vi "get_erbumen_sp_gonghao.vi"(2 "juese":string, 4 "gonghao":string) -> (0 "sp":string[][](array[string]), 1 "error":errorcluster caption="error out 10")   [LabVIEW 2017, in "Lib_code.lvlib"]
uses:
  Lib_code.lvlib
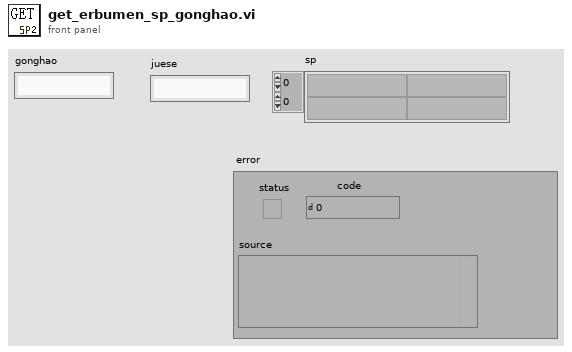
[diagram p1: front panel]
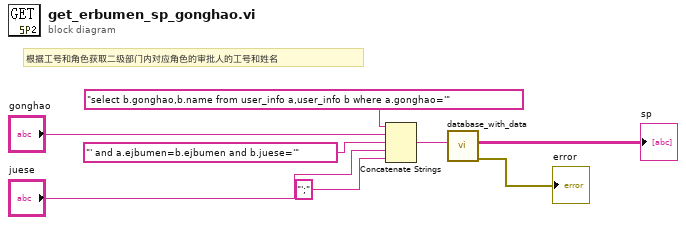
[diagram p0: block diagram]
diagram:
  # "根据工号和角色获取二级部门内对应角色的审批人的工号和姓名"
  n1 = Concatenate Strings("select b.gonghao,b.name from user_info a,user_info b where a.gonghao='" ("Command Text"), "gonghao", "' and a.ejbumen=b.ejbumen and b.juese='" ("字符串"), "juese", "';" ("字符串")) -> (w3:string)
  n2 = call "database_with_data.vi"("input"=w3) -> ("error"=→"error":errorcluster, "Data"=→"sp":string[][])  [unwired: 9 in]
